vi "StringArray Test.vi"() -> ()   [LabVIEW 2010]
uses:
  <vilib>/MDSplus/Library/Data/Array/StringArray/StringArray Create.vi
  <vilib>/MDSplus/Library/MDSplus.lvlib
panel:
  in  "String array in":string[](array[string])
  out "String array out":string[](array[string])
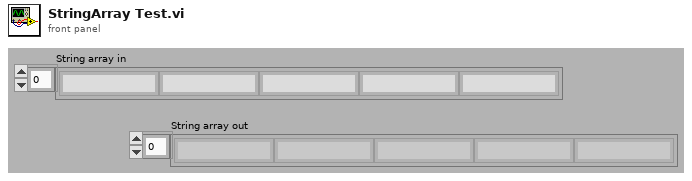
[diagram p1: front panel]
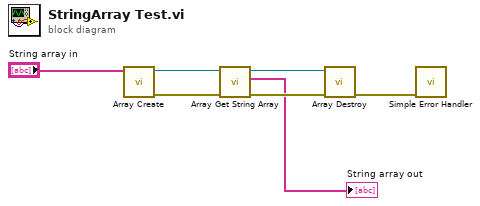
[diagram p0: block diagram]
diagram:
  n1 = call-poly <vilib>:"Array Create.vi"("String array in"="String array in") -> ("error out"=w6:errorcluster, "StringArray DVR out"=w7:refnum<data-value>)  [unwired: 9 in]
  n2 = call <vilib>:"Array Get String Array.vi"("error in (no error)"=w6, "Array DVR in"=w7) -> ("error out"=w4:errorcluster, "String array out"=→"String array out":string[], "Array DVR out"=w5:refnum<data-value>)  [unwired: 6 in, 1 out]
  n3 = call <vilib>:"Array Destroy.vi"("error in (no error)"=w4, "Array DVR in"=w5) -> ("error out"=w3:errorcluster)  [unwired: 9 in]
  n4 = call <vilib>:"Simple Error Handler.vi"("error in (no error)"=w3) -> ()  [unwired: 4 in, 5 out]
